vi "Rinocloud_HTTP_upload_file.vi"(6 "Extra metadata array":T1(array[cluster])=[{"Attribute"="", "Value"="", "Data type"=enum."<null>"}], 7 "Parent ID":string="name", 8 "Notes":string, 9 "Tags":string, 10 "Name":string, 11 "Path":path) -> (0 "Saved":bool, 1 "body":string, 2 "headers":string, 3 "Path out":path, 4 "ID":i32)   [LabVIEW 2013]
uses:
  Rinocloud_global_variable.vi
  <vilib>/httpClient/POSTFile.vi
  <vilib>/httpClient/LabVIEWHTTPClient.lvlib
panel:
  out "error out 2":errorcluster
  out "error out":errorcluster
  out "tmp file name":string
  out "JSON payload":string
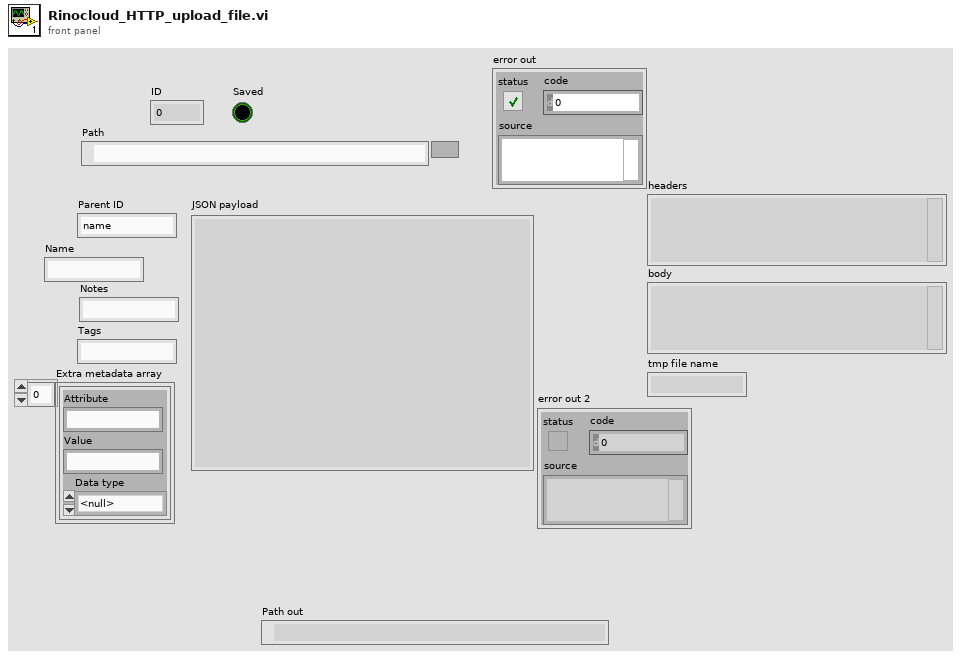
[diagram p1: front panel]
types:
  T1 = cluster{"Attribute":string, "Value":string, "Data type":enum16{"Numeric", "String", "1D array of strings", "1D array of doubles", "Data JSON string", "<null>"}}[]
  T2 = cluster{"Name":string, "Notes":string, "Tags":string}
  T3 = typedef "LabVIEWHTTPClient.lvlib/ClientHandle.ctl" = refnum<k1>
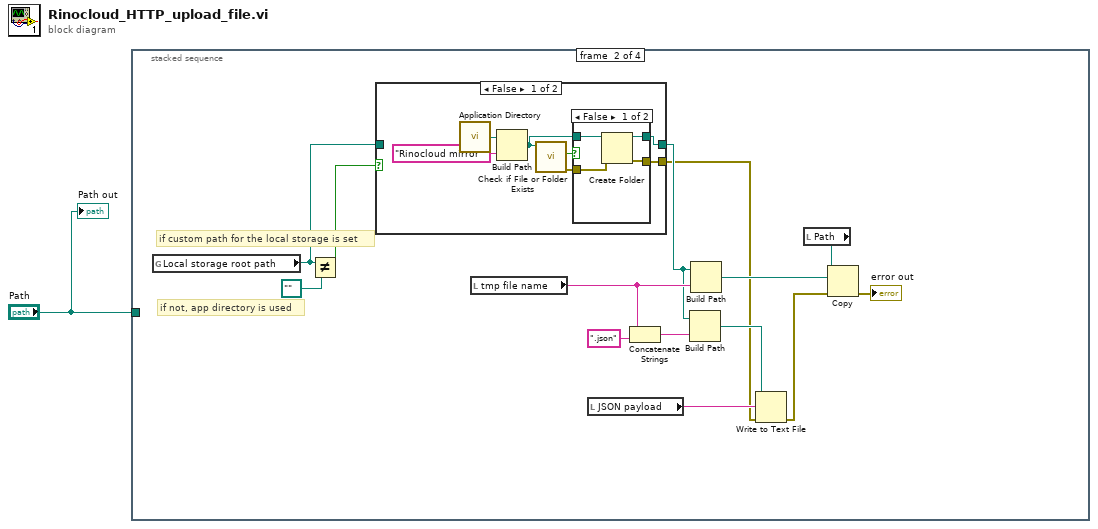
[diagram p0: block diagram]
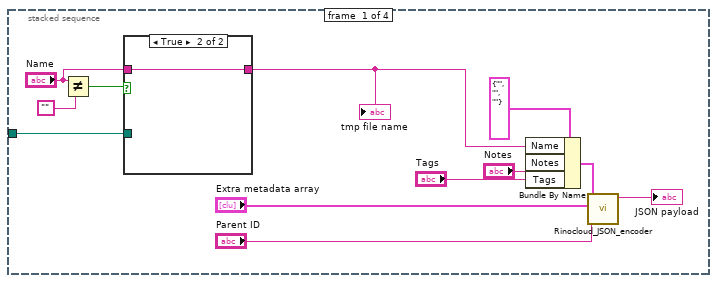
[diagram p2: hidden frame]
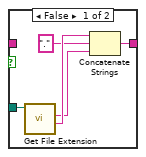
[diagram p3: hidden frame]
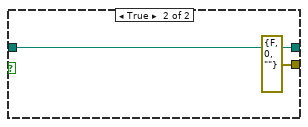
[diagram p5: hidden frame]
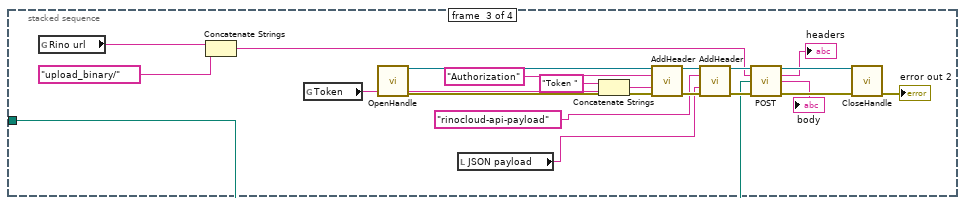
[diagram p6: hidden frame]
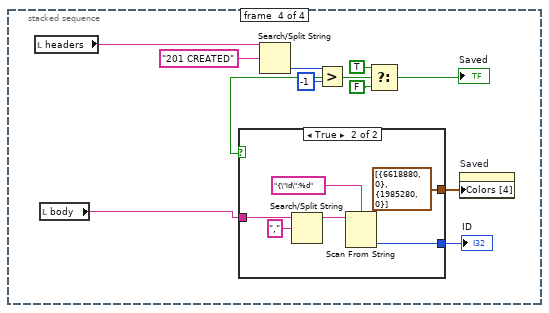
[diagram p7: hidden frame]
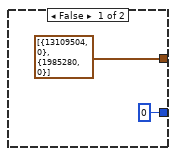
[diagram p8: hidden frame]
diagram:
  n1 = stacked-sequence {
    tunnel: "Path" -> [w2 _ w51 _]
    frame #0 {
      n2 = Not Equal?(x="Name", y="") -> (x != y?=w5:bool)
      n3 = case shown="True" w5 {
        tunnel: [w17 w19] -> w3
        tunnel: "Name" -> [_ w19]
        tunnel: w2 -> [w18 _]
        frame False {
          n4 = call <vilib>:"Get File Extension.vi"("file"=w18) -> ("filename without extension"=w16:string, "lowercase file extension"=w14:string)  [unwired: 7 in, 2 out]
          n5 = Concatenate Strings(w16, "." ("string"), w14) -> (w17:string)
        }
        frame True {
        }
      }
      "tmp file name" <- w3
      n6 = Bundle By Name(cluster=T2 {"Name"="", "Notes"="", "Tags"=""} ("Metadata"), "Name"=w3, "Notes"="Notes", "Tags"="Tags") -> (w9:T2)
      n7 = call "Rinocloud_JSON_encoder.vi"("parent ID"="Parent ID", "Extra metadata array"="Extra metadata array", "Metadata"=w9) -> ("JSON payload"=→"JSON payload":string)  [unwired: 8 in]
    }
    frame #1 {
      # "if not, app directory is used"
      # "if custom path for the local storage is set"
      n8 = global read "Rinocloud_global_variable.vi" "Local storage root path"() -> (w22:path)
      n9 = Not Equal?(x=w22, y=path "") -> (x != y?=w23:bool)
      n10 = case shown="False" w23 {
        tunnel: w22 -> [_ w48]
        tunnel: [w35 w48] -> w21
        tunnel: [w34 errorcluster {"status"=FALSE, "code"=0, "source"=""} ("error out")] -> w20
        frame False {
          n11 = call <vilib>:"Application Directory.vi"() -> ("Application Directory"=w36:path)
          n12 = Build Path(base path=w36, name or relative path="Rinocloud mirror") -> (appended path=w39:path)
          n13 = call <vilib>:"Check if File or Folder Exists.vi"("path"=w39) -> ("error out"=w40:errorcluster, "file or folder exists?"=w38:bool)  [unwired: 8 in, 1 out]
          n14 = case shown="False" w38 {
            tunnel: [w41 w46] -> w35
            tunnel: w39 -> [w44 w46]
            tunnel: w40 -> [w43 w45]
            tunnel: [w42 w45] -> w34
            frame False {
              n15 = Create Folder(path (use dialog)=w44, error in=w43) -> (created path=w41:path, error out=w42:errorcluster)  [unwired: 1 in, 1 out]
            }
            frame True {
            }
          }
        }
        frame True {
        }
      }
      n16 = local read "tmp file name"() -> (w29:string)
      n17 = local read "JSON payload"() -> (w30:string)
      n18 = Concatenate Strings(w29, ".json" ("string")) -> (w27:string)
      n19 = Build Path(base path=w21, name or relative path=w27) -> (appended path=w26:path)
      n20 = Build Path(base path=w21, name or relative path=w29) -> (appended path=w31:path)
      n21 = Write to Text File(file (use dialog)=w26, text=w30, error in=w20) -> (error out=w25:errorcluster)  [unwired: 1 in, 2 out]
      n22 = local read "Path"() -> (w32:path)
      n23 = Copy(8:w25, 10:w31, 11:w32) -> (0:→"error out":errorcluster)  [unwired: 2 in, 2 out]
    }
    frame #2 {
      n24 = global read "Rinocloud_global_variable.vi" "Rino url"() -> (w54:string)
      n25 = Concatenate Strings(w54, "upload_binary/" ("Combo Box 2")) -> (w52:string)
      n26 = global read "Rinocloud_global_variable.vi" "Token"() -> (w67:string)
      n27 = call <vilib>:"OpenHandle.vi"() -> ("client handle out"=w61:T3, "error out"=w64:errorcluster)  [unwired: 14 in]
      n28 = local read "JSON payload"() -> (w50:string)
      n29 = Concatenate Strings("Token " ("value"), w67) -> (w63:string)
      n30 = call <vilib>:"AddHeader.vi"("client handle"=w61, "header"="Authorization" ("url"), "value"=w63, "error in (no error)"=w64) -> ("client handle out"=w59:T3, "error out"=w65:errorcluster)  [unwired: 10 in]
      n31 = call <vilib>:"AddHeader.vi"("client handle"=w59, "header"="rinocloud-api-payload" ("value"), "value"=w50, "error in (no error)"=w65) -> ("client handle out"=w58:T3, "error out"=w66:errorcluster)  [unwired: 10 in]
      n32 = call-poly <vilib>:"POST.vi"("client handle"=w58, "url"=w52, "file"=w51, "error in (no error)"=w66) -> ("client handle out"=w68:T3, "headers"=→"headers":string, "body"=→"body":string, "error out"=w69:errorcluster)  [unwired: 8 in]
      n33 = call <vilib>:"CloseHandle.vi"("client handle"=w68, "error in (no error)"=w69) -> ("error out"=→"error out 2":errorcluster)  [unwired: 13 in]
    }
    frame #3 {
      n34 = local read "headers"() -> (w71:string)
      n35 = local read "body"() -> (w70:string)
      n36 = Search/Split String(string=w71, search string/char (-)="201 CREATED") -> (offset of match=w79:i32)  [unwired: 1 in, 2 out]
      n37 = Greater?(x=w79, y=-1) -> (0:w77:bool)
      n38 = Select(t=TRUE, s=w77, f=FALSE) -> (s? t:f=w74:bool)
      "Saved" <- w74
      n39 = case shown="True" w74 {
        tunnel: w70 -> [_ w88]
        tunnel: [0 w84] -> w73
        tunnel: [cluster{u32, u32}[] [{13109504, 0}, {1985280, 0}] ("Colors [4]") cluster{u32, u32}[] [{6618880, 0}, {1985280, 0}] ("Colors [4]")] -> w72
        frame False {
        }
        frame True {
          n40 = Search/Split String(string=w88, search string/char (-)=",") -> (substring before match=w86:string)  [unwired: 1 in, 2 out]
          n41 = Scan From String(format string="{\"id\":%d", input string=w86) -> (output 1=w84:i32)  [unwired: 3 in, 3 out]
        }
      }
      "ID" <- w73
      n42 = property on="Saved" class="Bool (strict)"("Colors [4]"=w72) -> ()  [unwired: 2 in, 2 out]
    }
  }
  "Path out" <- "Path"
